vi "PrintUserData.vi"(7 "Path":path=path "C:/LabViewTesty", 9 "Colors 4":u32[](array[colorbox])=[11796480, 37103, 40712, 16770816, 11796658, 4210752], 10 "Data:":string[](array[string]), 11 "Pie Chart All data \nto user data":picture) -> ()   [LabVIEW 2014]
panel:
  out "User data":T1={"Pie Chart All data \nto user data"=bytes[270], "Data:"=[], "Colors 4"=[11796480, 37103, 40712, 16770816, 11796658, 4210752], "Date"="", "Time"=""}
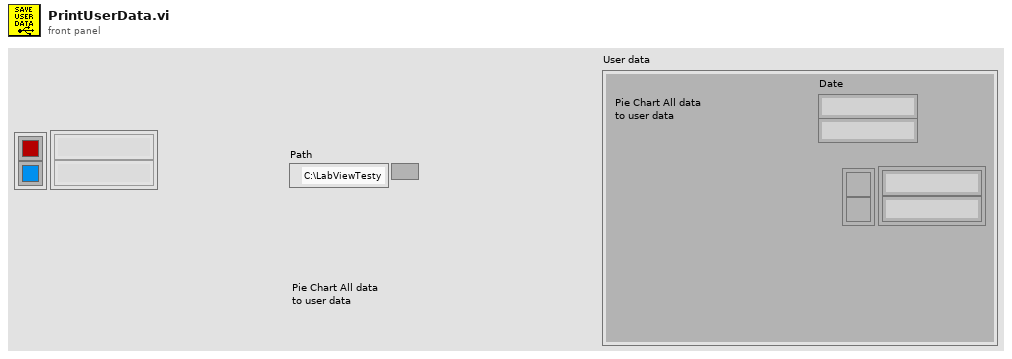
[diagram p1: front panel]
types:
  T1 = cluster{"Pie Chart All data \nto user data":picture, "Data:":string[], "Colors 4":u32[], "Date":string, "Time":string}
  T2 = typedef "imagedata.ctl" = cluster{"image type":i32, "image depth":i32, "image":u8[], "mask":u8[], "colors":u32[], "Rectangle":cluster{"left":i16, "top":i16, "right":i16, "bottom":i16}}
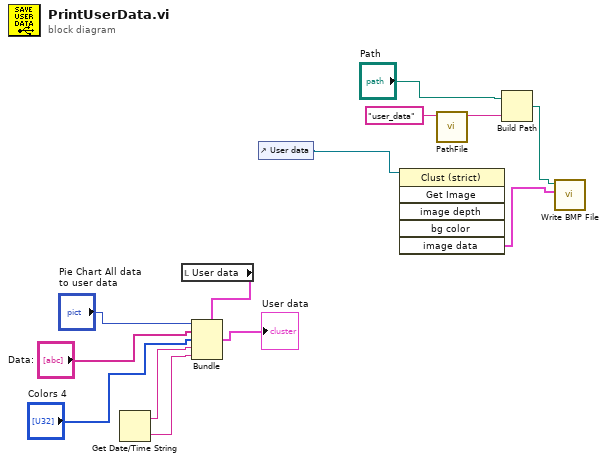
[diagram p0: block diagram]
diagram:
  n1 = Get Date/Time String() -> (date string=w3:string, time string=w2:string)  [unwired: 3 in]
  n2 = local read "User data"() -> (w8:T1)
  n3 = Bundle(cluster=w8, "Pie Chart All data \nto user data"="Pie Chart All data \nto user data", "Data:"="Data:", "Colors 4"="Colors 4", "Date"=w3, "Time"=w2) -> (→"User data":T1)
  n4 = control-ref of="User data"() -> (w1:refnum<vi>)
  n5 = invoke class="Clust (strict)" method="Get Image"(reference=w1) -> ("image data"=w13:T2)  [unwired: 5 in, 5 out]
  n6 = call "PathFile.vi"("NameFile"="user_data") -> ("stringNameFile"=w9:string)  [unwired: 10 in]
  n7 = Build Path(base path="Path", name or relative path=w9) -> (appended path=w12:path)
  n8 = call <vilib>:"Write BMP File.vi"("image data"=w13, "path to BMP file"=w12) -> ()  [unwired: 8 in, 2 out]
